vi "plink_sysE.vi"() -> ()   [LabVIEW 2020]
panel:
  out "error out":errorcluster
  in  "expected output size  (4096)":u32
  in  "standard input":string
  in  "working directory":path=path ""
  in  "run minimized? (F)":bool=TRUE
  in  "command line":string
  in  "wait until completion? (T)":bool=TRUE
  out "return code":i32
  out "standard error":string
  out "standard output":string
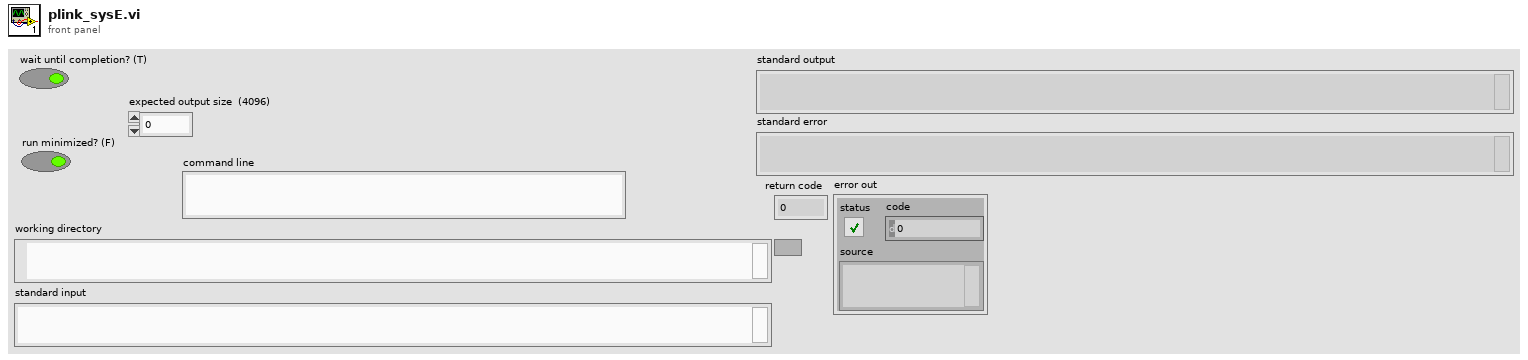
[diagram p1: front panel]
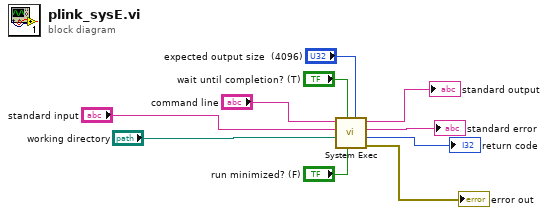
[diagram p0: block diagram]
diagram:
  n1 = call <vilib>:"System Exec.vi"("expected output size  (4096)"="expected output size  (4096)", "run minimized? (F)"="run minimized? (F)", "wait until completion? (T)"="wait until completion? (T)", "working directory"="working directory", "standard input"="standard input", "command line"="command line") -> ("error out"=→"error out":errorcluster, "return code"=→"return code":i32, "standard error"=→"standard error":string, "standard output"=→"standard output":string)  [unwired: 2 in]
